vi "Initialize Sections.vi"(0 "Device Configuration Data In":T4 {"Current Section Ref" format="%.0x"; "simTC Section Refs" format="%.0x"; "Voltage Section Ref" format="%.0x"; "Custom Device Ref" format="%.0x"}, 1 "Channel Data In":T1 {"Device Chan Total" max=32 step=1; "Thermocouple"."Temperature Units" items=["Celcius", "Fahrenheit", "Kelvin", "Rankine", "Volts"]; "Thermocouple"."Thermocouple Type" items=["J", "K", "T", "E", "N", "B", "R", "S", "Raw Voltage"]}, 3 "error in (no error)":errorcluster) -> (7 "Device Configuration Data  Out":T4 {"Current Section Ref" format="%.0x"; "simTC Section Refs" format="%.0x"; "Voltage Section Ref" format="%.0x"; "Custom Device Ref" format="%.0x"}, 8 "Channel Data Out":T1 {"Device Chan Total" max=32 step=1; "Thermocouple"."Temperature Units" items=["Celcius", "Fahrenheit", "Kelvin", "Rankine", "Volts"]; "Thermocouple"."Thermocouple Type" items=["J", "K", "T", "E", "N", "B", "R", "S", "Raw Voltage"]}, 10 "error Out (no error)":errorcluster)   [LabVIEW 2011, in "Simulated Thermocouple Custom Device.lvlib"]
uses:
  Simulated Thermocouple Custom Device.lvlib
  Device Config data.ctl
  <vilib>/NI Veristand/Custom Device API/Custom Device Item Ref.ctl
  New Channel Data.ctl
  TC Selector.ctl
  TC Unit Selector.ctl
  simTC Global GUIDs.vi
  <vilib>/NI Veristand/Custom Device API/Custom Device API.lvlib
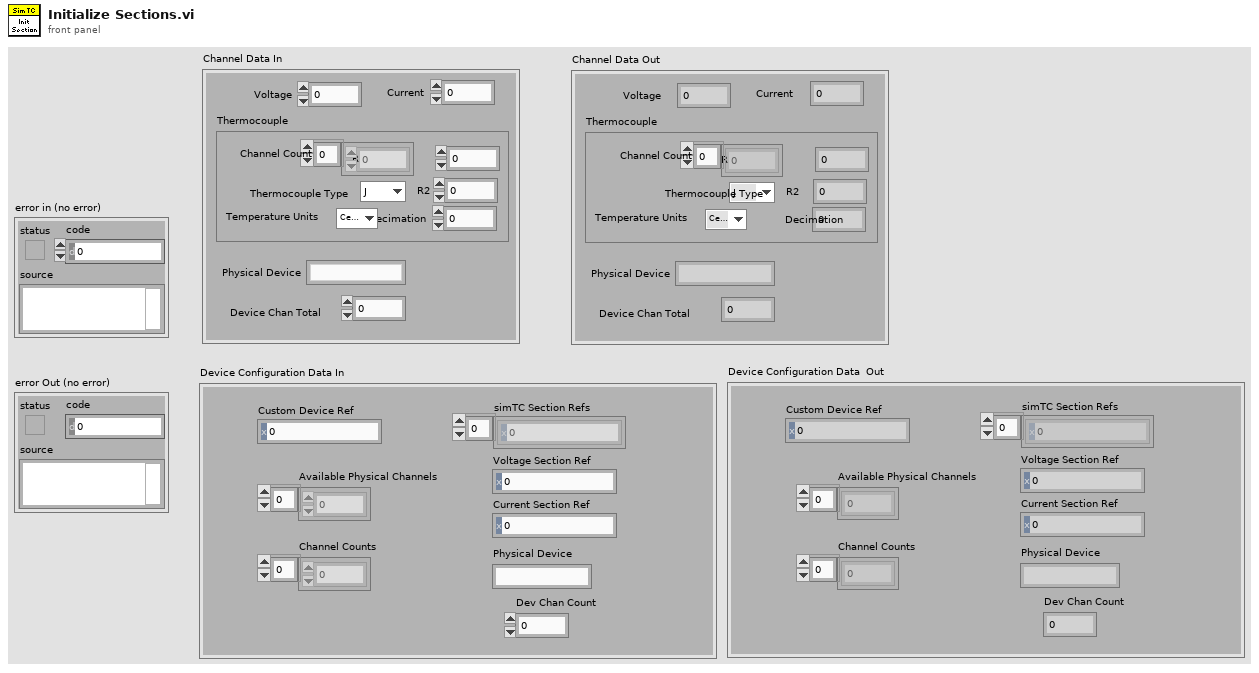
[diagram p1: front panel]
types:
  T1 = typedef "Simulated Thermocouple Custom Device.lvlib/New Channel Data.ctl" = cluster{"Voltage":u32, "Current":u32, "Thermocouple":cluster{"R1":dbl, "R2":dbl, "Decimation":u32, "Thermocouple Type":T2, "Temperature Units":T3, "Channel Count":u32[]}, "Physical Device":string, "Device Chan Total":u32}
  T2 = typedef "Simulated Thermocouple Custom Device.lvlib/TC Selector.ctl" = u16
  T3 = typedef "Simulated Thermocouple Custom Device.lvlib/TC Unit Selector.ctl" = u16
  T4 = typedef "Simulated Thermocouple Custom Device.lvlib/Device Config data.ctl" = cluster{"Custom Device Ref":T5, "Voltage Section Ref":T5, "simTC Section Refs":T5[], "Current Section Ref":T5, "Physical Device":string, "Available Physical Channels":i32[], "Channel Counts":u32[], "Dev Chan Count":u32}
  T5 = typedef "Custom Device API.lvlib/Custom Device Item Ref.ctl" = u64
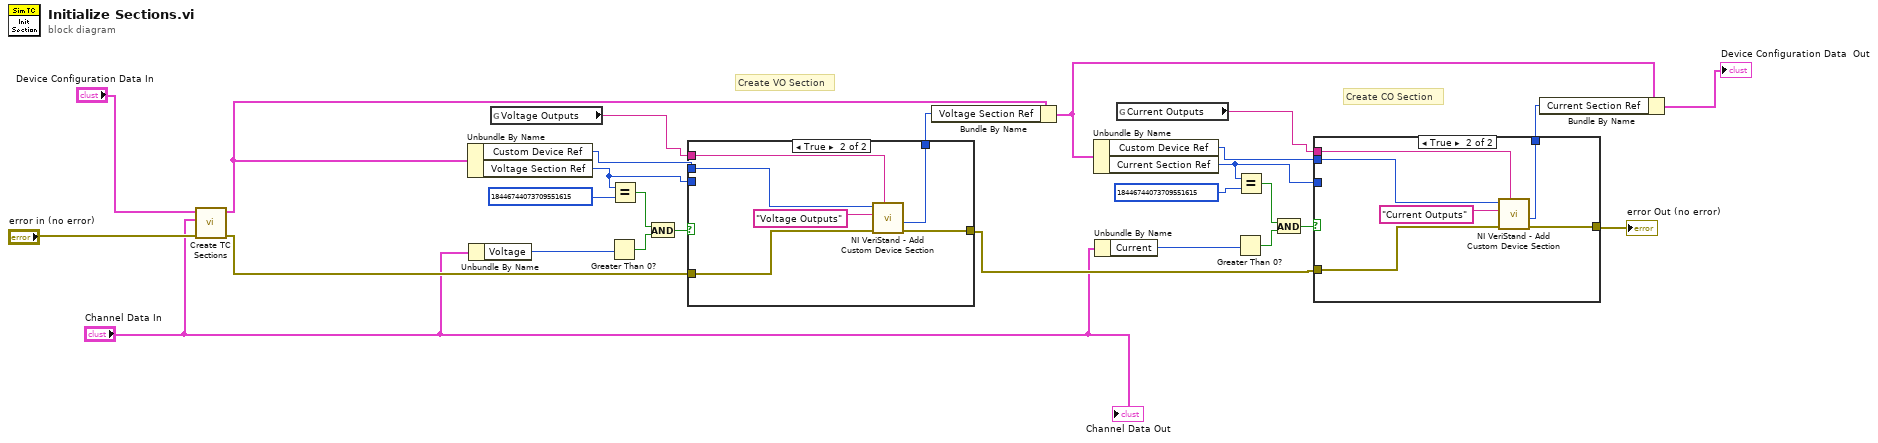
[diagram p0: block diagram]
diagram:
  # "Create CO Section"
  # "Create VO Section"
  n1 = call "Create TC Sections.vi"("error in (no error)"="error in (no error)", "Channel Data In"="Channel Data In", "Device Configuration Data In in"="Device Configuration Data In") -> ("error out"=w19:errorcluster, "Device Configuration Data In out"=w5:T4)  [unwired: 7 in]
  n2 = Unbundle By Name(w5) -> ("Custom Device Ref"=w21:T5, "Voltage Section Ref"=w7:T5)
  n3 = Unbundle By Name("Channel Data In") -> ("Voltage"=w22:u32)
  n4 = global read "simTC Global GUIDs.vi" "Voltage Outputs"() -> (w20:string)
  n5 = Greater Than 0?(x=w22) -> (x > 0?=w23:bool)
  n6 = Equal?(x=w7, y=T5 18446744073709551615) -> (x = y?=w24:bool)
  n7 = And(x=w24, y=w23) -> (x .and. y?=w25:bool)
  n8 = case shown="True" w25 {
    tunnel: w21 -> [_ w35]
    tunnel: w20 -> [_ w34]
    tunnel: w19 -> [w29 w33]
    tunnel: [w29 w31] -> w11
    tunnel: [w28 w30] -> w8
    tunnel: w7 -> [w28 _]
    frame False {
    }
    frame True {
      n9 = call <vilib>:"NI VeriStand - Add Custom Device Section.vi"("GUID (Default Section)"=w34, "error in (no error)"=w33, "Section Name"="Voltage Outputs", "Parent Ref in"=w35) -> ("error out"=w31:errorcluster, "Section Ptr"=w30:T5)  [unwired: 4 in, 2 out]
    }
  }
  n10 = Bundle By Name(cluster=w5, "Voltage Section Ref"=w8) -> (w3:T4)
  n11 = Unbundle By Name(w3) -> ("Custom Device Ref"=w17:T5, "Current Section Ref"=w6:T5)
  n12 = Unbundle By Name("Channel Data In") -> ("Current"=w16:u32)
  n13 = global read "simTC Global GUIDs.vi" "Current Outputs"() -> (w18:string)
  n14 = Greater Than 0?(x=w16) -> (x > 0?=w15:bool)
  n15 = Equal?(x=w6, y=T5 18446744073709551615) -> (x = y?=w14:bool)
  n16 = And(x=w14, y=w15) -> (x .and. y?=w13:bool)
  n17 = case shown="True" w13 {
    tunnel: w17 -> [_ w43]
    tunnel: w18 -> [_ w42]
    tunnel: w11 -> [w37 w41]
    tunnel: [w37 w39] -> w10
    tunnel: w6 -> [w36 _]
    tunnel: [w36 w38] -> w2
    frame False {
    }
    frame True {
      n18 = call <vilib>:"NI VeriStand - Add Custom Device Section.vi"("GUID (Default Section)"=w42, "error in (no error)"=w41, "Section Name"="Current Outputs", "Parent Ref in"=w43) -> ("error out"=w39:errorcluster, "Section Ptr"=w38:T5)  [unwired: 4 in, 2 out]
    }
  }
  "error Out (no error)" <- w10
  n19 = Bundle By Name(cluster=w3, "Current Section Ref"=w2) -> (→"Device Configuration Data  Out":T4)
  "Channel Data Out" <- "Channel Data In"
